vi "oauth2-from_oauth1.vi"(8 "error in (no error)":errorcluster, 10 "app_secret":string, 11 "app_key":string) -> (0 "error out":errorcluster, 3 "oauth2_token":string)   [LabVIEW 2015, in "lv-dropbox.lvlib"]
uses:
  lv-dropbox.lvlib
  private/_controls/content_type.ctl
  <vilib>/httpClient/POSTBuffer.vi
  <vilib>/httpClient/LabVIEWHTTPClient.lvlib
panel:
  in  "code_verifier":string
  in  "authorization_code":string
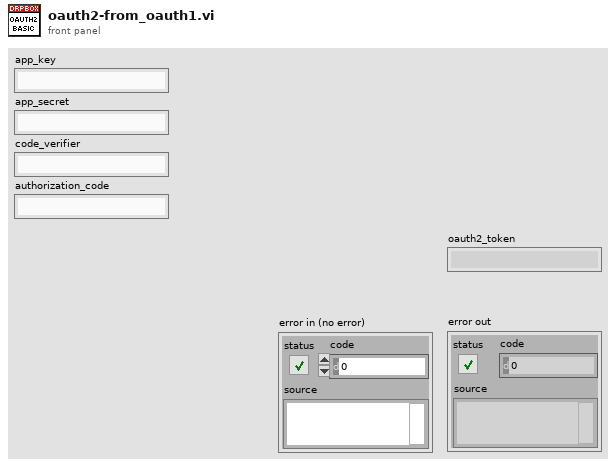
[diagram p1: front panel]
types:
  T1 = typedef "lv-dropbox.lvlib/content_type.ctl" = enum16{"<content_type>", "application/json", "application/octet-stream", "application/x-www-form-urlencoded"}
  T2 = typedef "LabVIEWHTTPClient.lvlib/ClientHandle.ctl" = refnum<k1>
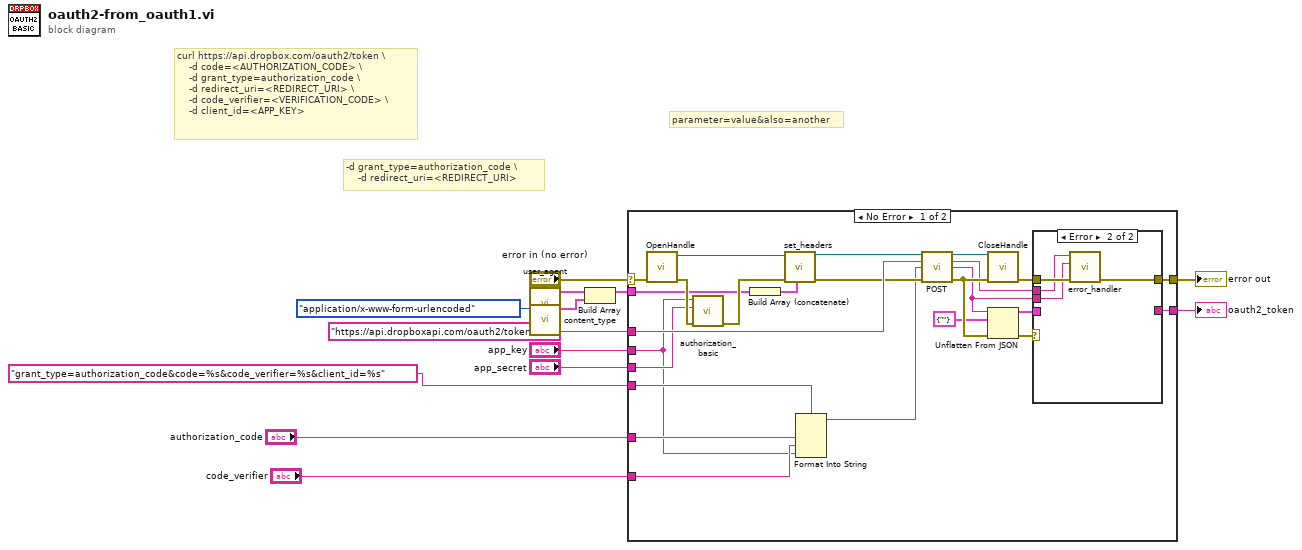
[diagram p0: block diagram]
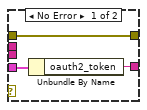
[diagram p2: hidden frame]
diagram:
  # "curl https://api.dropbox.com/oauth2/token \\\n    -d code=<AUTHORIZATION_CODE> \\\n    -d grant_type=authorization_code \\\n    -d redirect_uri=<REDIRECT_URI> \\\n    -d code_verifier=<VERIFICATION_CODE> \\\n    -d client_id=<APP_KEY>"
  # "parameter=value&also=another"
  # "-d grant_type=authorization_code \\\n    -d redirect_uri=<REDIRECT_URI>"
  n1 = call "user_agent.vi"() -> ("header"=w10:cluster{"header":string, "value":string})  [unwired: 11 in]
  n2 = call "content_type.vi"("content_type"=content_type."application/x-www-form-urlencoded") -> ("header"=w11:cluster{"header":string, "value":string})  [unwired: 10 in]
  n3 = Build Array(w10, w11) -> (w12:cluster{"header":string, "value":string}[])
  n4 = case shown="No Error" "error in (no error)" {
    selector: "error in (no error)" -> [w31 w46]
    tunnel: "https://api.dropboxapi.com/oauth2/token" ("url") -> [w35 _]
    tunnel: w12 -> [w30 _]
    tunnel: [w25 w46] -> w8
    tunnel: "app_key" -> [w14 _]
    tunnel: "app_secret" -> [w21 _]
    tunnel: [w20 _] -> w5
    tunnel: "authorization_code" -> [w18 _]
    tunnel: "grant_type=authorization_code&code=%s&code_verifier=%s&client_id=%s" -> [w16 _]
    tunnel: "code_verifier" -> [w15 _]
    frame No Error {
      n5 = call <vilib>:"OpenHandle.vi"("error in (no error)"=w31) -> ("client handle out"=w32:T2, "error out"=w38:errorcluster)  [unwired: 13 in]
      n6 = call "authorization_basic.vi"("error in (no error)"=w38, "password"=w21, "username"=w14) -> ("error out"=w37:errorcluster)  [unwired: 7 in, 1 out]
      n7 = Build Array (concatenate)(w30) -> (w22:cluster{"header":string, "value":string}[])
      n8 = call "set_headers.vi"("header_value []"=w22, "error in (no error)"=w37, "client_handle in"=w32) -> ("error out"=w19:errorcluster, "client_handle out"=w29:T2)  [unwired: 7 in]
      n9 = Format Into String(format string=w16, w18, w15, w14) -> (resulting string=w17:string)  [unwired: 2 in, 1 out]
      n10 = call-poly <vilib>:"POST.vi"("client handle"=w29, "url"=w35, "buffer"=w17, "error in (no error)"=w19) -> ("client handle out"=w28:T2, "headers"=w24:string, "body"=w23:string, "error out"=w36:errorcluster)  [unwired: 8 in]
      n11 = call <vilib>:"CloseHandle.vi"("client handle"=w28, "error in (no error)"=w36) -> ("error out"=w26:errorcluster)  [unwired: 13 in]
      n12 = Unflatten From JSON(JSON string=w23, type and defaults=cluster{"oauth2_token":string} {"oauth2_token"=""} ("value"), error in (no error)=w36) -> (value=w33:cluster{"oauth2_token":string}, error out=w27:errorcluster)  [unwired: 4 in]
      n13 = case shown="Error" w27 {
        tunnel: w33 -> [w40 _]
        tunnel: w26 -> [w41 w45]
        tunnel: [w41 w42] -> w25
        tunnel: w24 -> [_ w44]
        tunnel: w23 -> [_ w43]
        tunnel: [w39 _] -> w20
        frame No Error {
          n14 = Unbundle By Name(w40) -> ("oauth2_token"=w39:string)
        }
        frame Error {
          n15 = call "error_handler.vi"("error in (no error)"=w45, "body"=w43, "headers"=w44) -> ("error out"=w42:errorcluster)  [unwired: 8 in]
        }
      }
    }
    frame Error {
    }
  }
  "error out" <- w8
  "oauth2_token" <- w5
